vi "set_default_speed_by_name.vi"(8 "error in (no error)":errorcluster caption="错误输入（无错误）", 9 "speed":i32, 10 "name":string, 11 "MotorSystem 输入":refnum<class "MotorSystem.lvclass">) -> (0 "error out":errorcluster caption="错误输出", 3 "MotorSystem 输出":refnum<class "MotorSystem.lvclass">)   [LabVIEW 2016, in "MotionControl_UFO_3DOF.lvlib" / "MotorSystem.lvclass"]
uses:
  <userlib>/MotionControl_UFO_3DOF/MotorSystem/MotorSystem.lvclass
  <userlib>/MotionControl_UFO_3DOF/MotorSystem/MotorSystem.lvclass/MotorSystem.ctl
  <userlib>/MotionControl_UFO_3DOF/OneMotion/OneMotion.lvclass
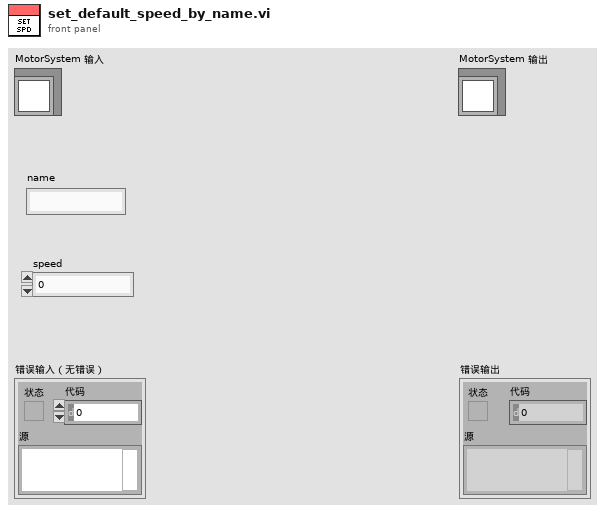
[diagram p1: front panel]
types:
  T1 = typedef "MotionControl_UFO_3DOF.lvlib/MotorSystem.lvclass/MotionCluster.ctl" = cluster{"OneMotion.lvclass":refnum<class "OneMotion.lvclass">, "connected?":bool, "default enabled?":bool, "enabled?":bool}
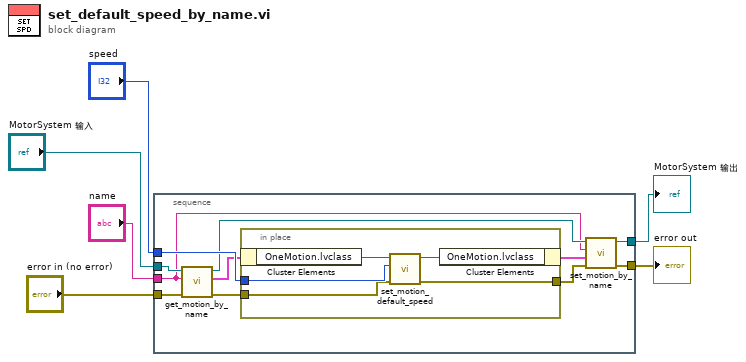
[diagram p0: block diagram]
diagram:
  n1 = stacked-sequence {
    tunnel: [w7] -> w6
    tunnel: [w9] -> w4
    tunnel: "MotorSystem 输入" -> [w17]
    tunnel: "error in (no error)" -> [w16]
    tunnel: "name" -> [w11]
    tunnel: "speed" -> [w15]
    frame #0 {
      n2 = call <userlib>:"get_motion_by_name.vi"("error in (no error)"=w16, "name"=w11, "MotorSystem in"=w17) -> ("error out"=w14:errorcluster, "motion cluster"=w13:T1, "MotorSystem out"=w12:refnum<class "MotorSystem.lvclass">)  [unwired: 6 in]
      n3 = in-place {
        in-place-border: w15 -> [w22]
        in-place-border: w14 -> [w21]
        in-place-border: [w20] -> w8
        n4 = in-place-cluster #1(w13) -> ("OneMotion.lvclass"=w19:refnum<class "OneMotion.lvclass">)
        n5 = call <userlib>:"set_motion_default_speed.vi"("error in (no error)"=w21, "default speed"=w22, "OneMotion 输入"=w19) -> ("error out"=w20:errorcluster, "OneMotion 输出"=w18:refnum<class "OneMotion.lvclass">)  [unwired: 7 in]
        n6 = in-place-cluster #1("OneMotion.lvclass"=w18) -> (w10:T1)
      }
      n7 = call <userlib>:"set_motion_by_name.vi"("error in (no error)"=w8, "簇"=w10, "name"=w11, "MotorSystem输入"=w12) -> ("error out"=w7:errorcluster, "MotorSystem输出"=w9:refnum<class "MotorSystem.lvclass">)  [unwired: 6 in]
    }
  }
  "error out" <- w6
  "MotorSystem 输出" <- w4
